vi "Get Generic Slave IOVars.vi"(8 "error in (no error)":errorcluster, 11 "ECAT Slave in":refnum<k21>="ni.var.io://localhost/EtherCAT Master/Device") -> (0 "error IO":errorcluster, 2 "ECAT Variablenobjekt":refnum<k21>[](array[refnum]), 3 "ECAT Slave out":refnum<k21>="ni.var.io:/")   [LabVIEW 2020, in "SEECD Engine.lvlib"]
uses:
  SEECD Engine.lvlib
  <resource>/objmgr/IndComECAT.rc
  <vilib>/NI VeriStand/Custom Device Tools/Custom Device Utility Library/Custom Device Utility Library.lvlib
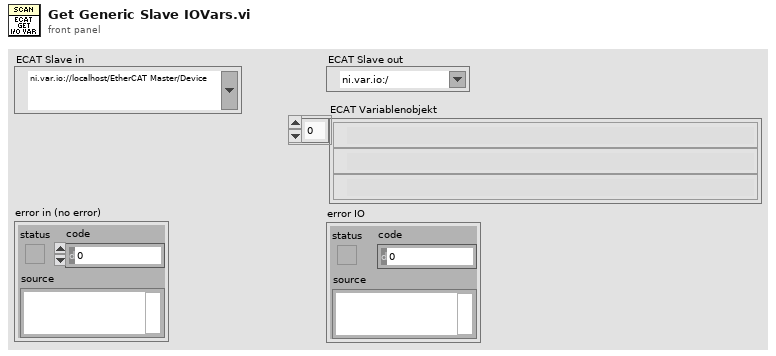
[diagram p1: front panel]
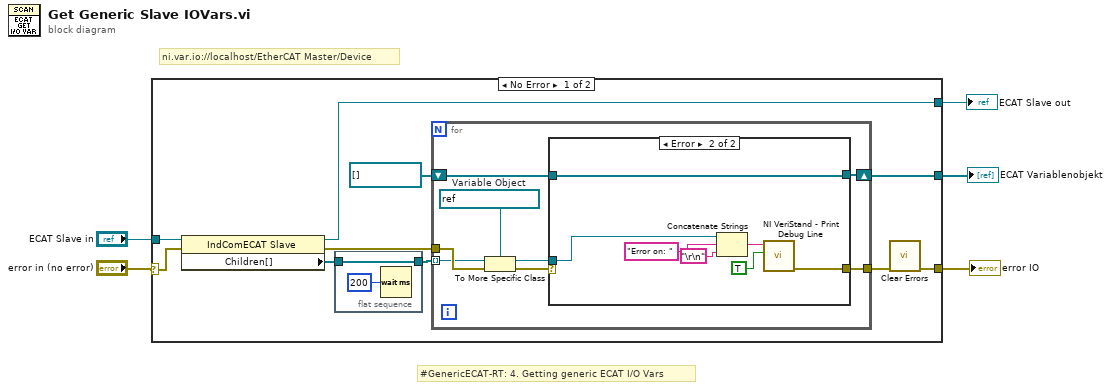
[diagram p0: block diagram]
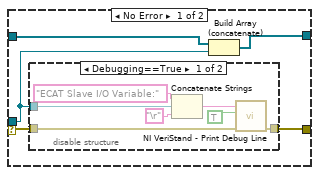
[diagram p2: hidden frame]
diagram:
  # "#GenericECAT-RT: 4. Getting generic ECAT I/O Vars"
  # "ni.var.io://localhost/EtherCAT Master/Device"
  n1 = case shown="No Error" "error in (no error)" {
    selector: "error in (no error)" -> [w12 w47]
    tunnel: [w15 w47] -> w1
    tunnel: "ECAT Slave in" -> [w14 w46]
    tunnel: [w13 w46] -> w4
    tunnel: [w6 _] -> w2
    frame No Error {
      n2 = property class="IndComECAT Slave"(reference=w14, error in=w12) -> (reference out=w13:refnum<k21>, error out=w11:errorcluster, "Children[]"=w9:refnum<k21>[])
      n3 = flat-sequence {
        tunnel: w9 -> [w17]
        tunnel: [w17] -> w8
        frame #0 {
          n4 = Wait (ms)(milliseconds to wait=u32 200) -> ()  [unwired: 1 out]
        }
      }
      n5 = for {
        tunnel: w8 -> [w21] mode=indexing
        tunnel: w11 -> [w25]
        tunnel: [w24] -> w10
        shift-right: [w20] -> w6
        shift-left: refnum<k21>[] [] -> [w19]
        w18 = refnum<k21> refnum  # Variable Object
        n6 = To More Specific Class(target class=w18, reference=w21, error in=w25) -> (specific class reference=w22:refnum<k21>, error out=w23:errorcluster)
        n7 = case shown="Error" w23 {
          selector: w23 -> [w26 _]
          tunnel: w22 -> [w28 w44]
          tunnel: [w27 w40] -> w24
          tunnel: [w29 w45] -> w20
          tunnel: w19 -> [w30 w45]
          frame No Error {
            n8 = disable-structure shown="Debugging==True" {
              disable-tunnel: w28 -> [w37 _]
              disable-tunnel: [w35 w38] -> w27
              disable-tunnel: w26 -> [w34 w38]
              frame condition #0 {
                n9 = Concatenate Strings("ECAT Slave I/O Variable:", w37, "\r") -> (w33:string)
                n10 = call <vilib>:"NI VeriStand - Print Debug Line.vi"("error in (no error)"=w34, "Add to log file? (F)"=TRUE, "Message"=w33) -> ("error out"=w35:errorcluster)  [unwired: 8 in]
              }
              frame condition #1 (active) {
              }
            }
            n11 = Build Array (concatenate)(w30, w28) -> (w29:refnum<k21>[])
          }
          frame Error {
            n12 = Concatenate Strings(w44, "Error on: ", "\r\n") -> (w41:string)
            n13 = call <vilib>:"NI VeriStand - Print Debug Line.vi"("Add to log file? (F)"=TRUE ("Add to log file? (T)"), "Message"=w41) -> ("error out"=w40:errorcluster)  [unwired: 9 in]
          }
        }
      }
      n14 = call <vilib>:"Clear Errors.vi"("error in (no error)"=w10) -> ("error out"=w15:errorcluster)  [unwired: 5 in, 1 out]
    }
    frame Error {
    }
  }
  "error IO" <- w1
  "ECAT Slave out" <- w4
  "ECAT Variablenobjekt" <- w2
